vi "cRIO Read Vendor Name.vi"(8 "error in (no error)":errorcluster, 11 "Refnum in":T1) -> (0 "error out":errorcluster, 2 "Vendor Name":string, 3 "Refnum out":T1)   [LabVIEW 2017, in "cRIODetectHW.lvlib"]
uses:
  <vilib>/addons/cRIODetectHW/cRIODetectHW.lvlib
  <vilib>/addons/cRIODetectHW/control/FPGARef.ctl
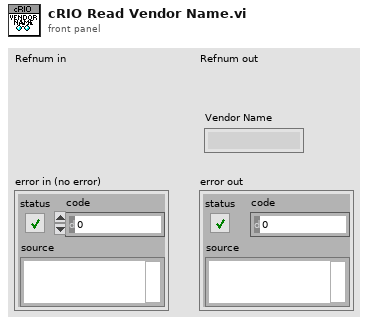
[diagram p1: front panel]
types:
  T1 = typedef "cRIODetectHW.lvlib/FPGARef.ctl" = refnum<k20>
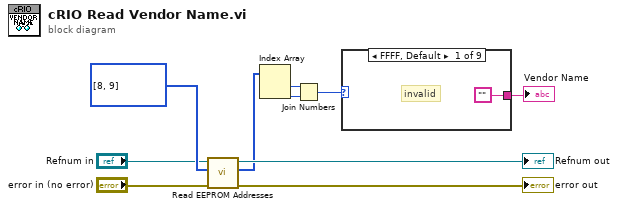
[diagram p0: block diagram]
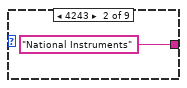
[diagram p2: hidden frame]
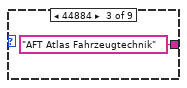
[diagram p3: hidden frame]
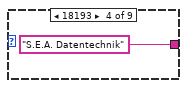
[diagram p4: hidden frame]
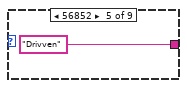
[diagram p5: hidden frame]
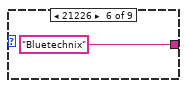
[diagram p6: hidden frame]
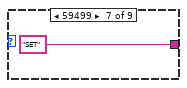
[diagram p7: hidden frame]
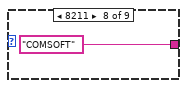
[diagram p8: hidden frame]
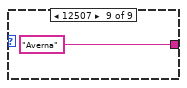
[diagram p9: hidden frame]
diagram:
  n1 = call <vilib>:"Read EEPROM Addresses.vi"("error in (no error)"="error in (no error)", "Addresses"=u16[] [8, 9], "Refnum in"="Refnum in") -> ("error out"=→"error out":errorcluster, "Data"=w3:u8[], "Refnum out"=→"Refnum out":T1)  [unwired: 6 in]
  n2 = Index Array(array=w3) -> (element #1=w5:u8, element #2=w4:u8)  [unwired: 2 in]
  n3 = Join Numbers(hi=w5, lo=w4) -> ((hi.lo)=w2:u16)
  n4 = case shown="FFFF, Default" w2 {
    tunnel: ["" "National Instruments" "AFT Atlas Fahrzeugtechnik" "S.E.A. Datentechnik" "Drivven" "Bluetechnix" "SET" "COMSOFT" "Averna"] -> w1
    frame 65535, Default {
      # "invalid"
    }
    frame 4243 {
    }
    frame 44884 {
    }
    frame 18193 {
    }
    frame 56852 {
    }
    frame 21226 {
    }
    frame 59499 {
    }
    frame 8211 {
    }
    frame 12507 {
    }
  }
  "Vendor Name" <- w1
